vi "get all FPGA resources.vi"(8 "error in (no error)":errorcluster, 11 "Item Ref in":T1 format="%.0x") -> (0 "error out":errorcluster, 2 "fpga resources":cluster{"fpga cd":T1, "resource":T2}[](array[cluster]) {"fpga cd" format="%.0x"}, 3 "Item Ref out":T1 format="%.0x")   [LabVIEW 2016, in "FPGA RM System Definition API.lvlib"]
doc: "Returns an array of all FPGA resources in the current System Definition"
uses:
  FPGA RM System Definition API.lvlib
  <vilib>/NI Veristand/Custom Device API/Custom Device Item Ref.ctl
  Types/fpga resource.ctl
  Types/Channel Type.ctl
  <vilib>/NI VeriStand/Custom Device API/Custom Device API.lvlib
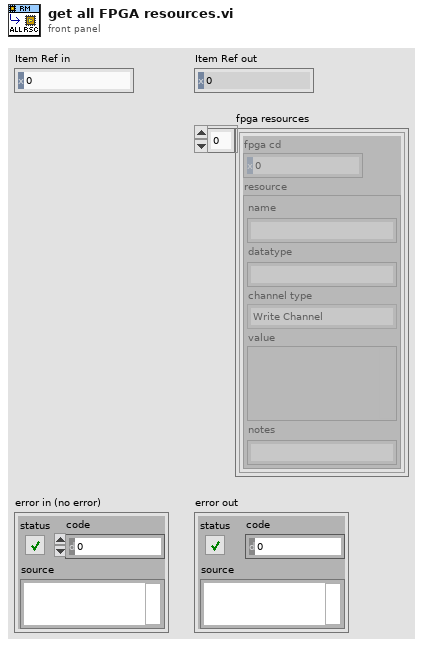
[diagram p1: front panel]
types:
  T1 = typedef "Custom Device API.lvlib/Custom Device Item Ref.ctl" = u64
  T2 = typedef "FPGA RM System Definition API.lvlib/fpga resource.ctl" = cluster{"name":string, "datatype":string, "channel type":T3, "value":variant, "notes":string}
  T3 = typedef "FPGA RM System Definition API.lvlib/Channel Type.ctl" = enum16{"Write Channel", "Read Channel", "Write Waveform", "Read Waveform"}
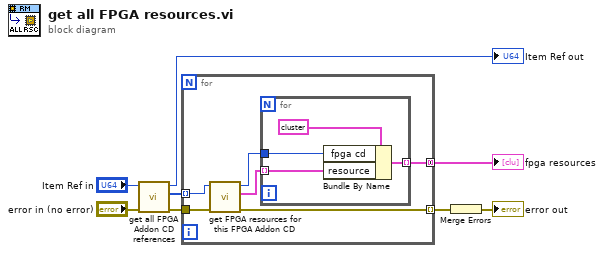
[diagram p0: block diagram]
diagram:
  n1 = call "get all FPGA Addon CD references.vi"("error in (no error)"="error in (no error)", "Item Ref in"="Item Ref in") -> ("error out"=w3:errorcluster, "FPGA Addon CD refs out"=w5:T1[], "Item Ref out"=→"Item Ref out":T1)  [unwired: 7 in]
  n2 = for {
    tunnel: w3 -> [w14]
    tunnel: w5 -> [w12] mode=indexing
    tunnel: [w13] -> w8 mode=indexing
    tunnel: [w9] -> w1 mode=concatenating
    n3 = call "get FPGA resources for this FPGA Addon CD.vi"("error in (no error)"=w14, "Item Ref in"=w12) -> ("error out"=w13:errorcluster, "fpga resources"=w11:T2[], "Item Ref out"=w10:T1)  [unwired: 6 in, 1 out]
    n4 = for {
      tunnel: w11 -> [w18] mode=indexing
      tunnel: w10 -> [w17]
      tunnel: [w15] -> w9 mode=indexing
      n5 = Bundle By Name(cluster=cluster{"fpga cd":T1, "resource":T2} {"fpga cd"=0, "resource"={"name"="", "datatype"="", "channel type"=enum."Write Channel", "value"=variant, "notes"=""}}, "fpga cd"=w17, "resource"=w18) -> (w15:cluster{"fpga cd":T1, "resource":T2})
    }
  }
  "fpga resources" <- w1
  n6 = Merge Errors(w8) -> (→"error out":errorcluster)
